vi "IDN.vi"(8 "error in (no error)":errorcluster, 11 "RP Communicator in":refnum<class "RP Communicator VISA.lvclass">) -> (0 "error out":errorcluster, 1 "Logic tag":u16, 2 "IDN response":u32=1 format="0x%x (%d)", 3 "RP Communicator out":refnum<class "RP Communicator VISA.lvclass">)   [LabVIEW 2016, in "RP Communicator VISA.lvclass"]
uses:
  RP Communicator VISA.lvclass
  RP Command.ctl
  RP Communicator VISA.lvclass/RP Communicator VISA.ctl
  RP Write Command VISA.vi
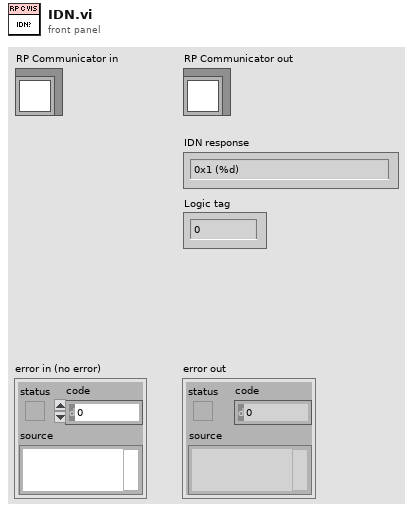
[diagram p1: front panel]
types:
  T1 = enum16{"big-endian, network order", "native, host order", "little-endian"}
  T2 = typedef "RP Command.ctl" = enum16{"Reset", "Read IDN", "Stop server", "Get status", "Get temperature", "Connect client", "Arm", "Software trigger", "Get whole buffer", "Get chunk", "System call", "Get config", "Set config", "Recieve data", "Play pattern", "Transmit data"}
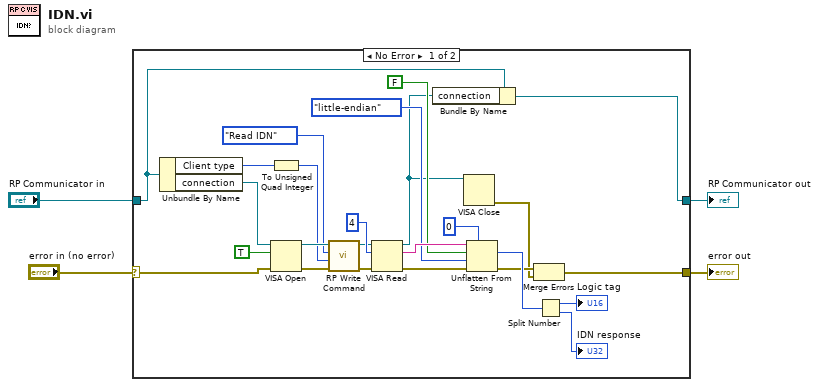
[diagram p0: block diagram]
diagram:
  n1 = case shown="No Error" "error in (no error)" {
    selector: "error in (no error)" -> [w29 w31]
    tunnel: [w12 w31] -> w3
    tunnel: [w24 w30] -> w1
    tunnel: "RP Communicator in" -> [w25 w30]
    frame No Error {
      n2 = Unbundle By Name(w25) -> ("Client type"=w26:enum16{"Control", "Reciever", "Transmitter"}, "connection"=w7:refnum<visa-resource-name>)
      n3 = To Unsigned Quad Integer(1:w26) -> (0:w22:u64)
      n4 = VISA Open(duplicate session (F)=TRUE, error in (no error)=w29, VISA resource name=w7) -> (VISA resource name=w27:refnum<visa-resource-name>, error out=w28:errorcluster)  [unwired: 2 in]
      n5 = call-poly "RP Write Command.vi"("Error In"=w28, "Command payload"=w22, "Command number"=RP_Command."Read IDN", "VISA resource"=w27) -> ("Error Out"=w14:errorcluster, "VISA resource out"=w15:refnum<visa-resource-name>)  [unwired: 5 in, 1 out]
      n6 = VISA Read(VISA resource name=w15, byte count=4 ("bytes to read"), error in (no error)=w14) -> (VISA resource name out=w6:refnum<visa-resource-name>, read buffer=w21:string, error out=w10:errorcluster)  [unwired: 1 out]
      n7 = Bundle By Name(cluster=w25, "connection"=w6) -> (w24:refnum<class "RP Communicator VISA.lvclass">)
      n8 = VISA Close(VISA resource name=w6) -> (error out=w11:errorcluster)  [unwired: 1 in]
      n9 = Unflatten From String(type=u32 0, binary string=w21, data includes array or string size? (T)=FALSE, byte order (0:big-endian, network order)=T1."little-endian", error in (no error)=w10) -> (value=w16:u32, error out=w13:errorcluster)  [unwired: 1 out]
      n10 = Merge Errors(w13, w11) -> (w12:errorcluster)
      n11 = Split Number(x=w16) -> (hi(x)=→"Logic tag":u16, lo(x)=→"IDN response":u16)
    }
    frame Error {
    }
  }
  "error out" <- w3
  "RP Communicator out" <- w1
